vi "Interpolate Real.vi"(6 "interpolation_degree":i32=1, 7 "method":i32(ring)=2 items=["nearest", "linear", "spline", "cubic Hermite", "Lagrange"], 9 "n":dbl[](array[numeric]), 11 "Y":dbl[](array[numeric])) -> (0 "N_interpolated":i32, 1 "n_interpolated":dbl[](array[numeric]), 3 "Y_interpolated":dbl[](array[numeric]))   [LabVIEW 2014]
uses:
  <vilib>/gmath/NI_Gmath.lvlib
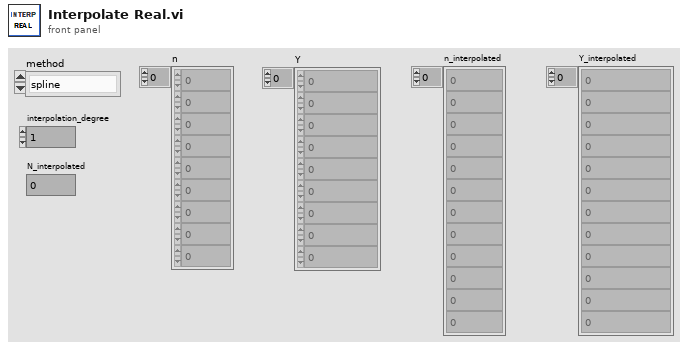
[diagram p1: front panel]
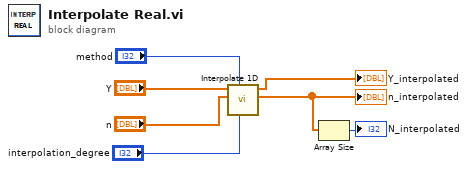
[diagram p0: block diagram]
diagram:
  n1 = call <vilib>:"Interpolate 1D.vi"("ntimes"="interpolation_degree", "method"="method", "X"="n", "Y"="Y") -> ("xi used"=w4:dbl[], "yi"=→"Y_interpolated":dbl[])  [unwired: 5 in, 1 out]
  "n_interpolated" <- w4
  n2 = Array Size(array=w4) -> (size(s)=→"N_interpolated":i32)
